vi "Remove Indentation.vi"(10 "levels to remove":i32, 11 "String in":string) -> (3 "String":string)   [LabVIEW 2013]
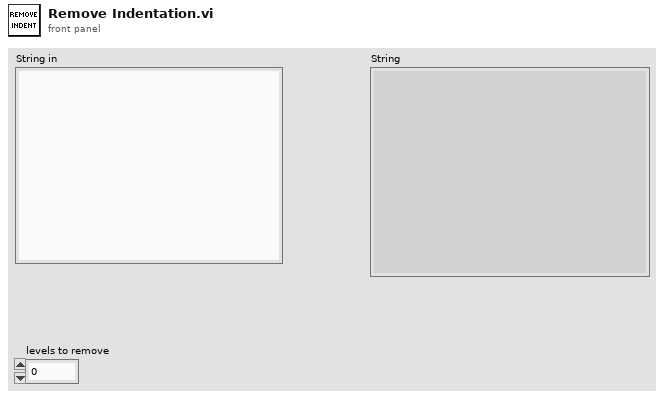
[diagram p1: front panel]
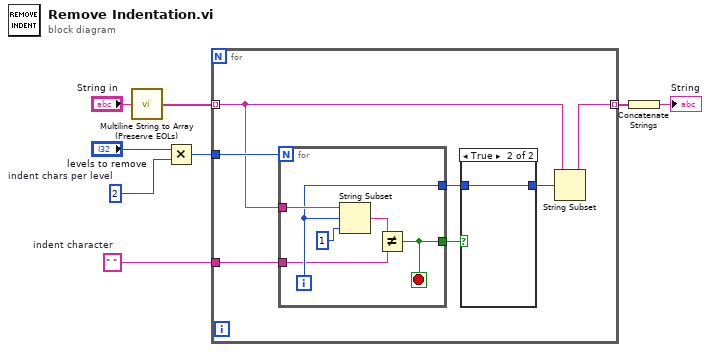
[diagram p0: block diagram]
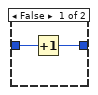
[diagram p2: hidden frame]
diagram:
  w1 = " "  # indent character
  w5 = 2  # indent chars per level
  n1 = call "Multiline String to Array (Preserve EOLs).vi"("Input String"="String in") -> ("Array"=w7:string[])
  n2 = Multiply(x="levels to remove", y=w5) -> (x*y=w4:i32)
  n3 = for {
    tunnel: w7 -> [w14] mode=indexing
    tunnel: w4 -> [w15]
    tunnel: [w13] -> w3 mode=indexing
    tunnel: w1 -> [w9]
    n4 = for {
      N: w15 -> [_]
      tunnel: w14 -> [w24]
      tunnel: [w21] -> w10
      tunnel: [w20] -> w12
      tunnel: w9 -> [w19]
      i -> [w21]
      stop <- w20 stop-if-true
      n5 = String Subset(string=w24, offset (0)=w21, length (rest)=1 ("length (rest)")) -> (substring=w22:string)
      n6 = Not Equal?(x=w22, y=w19) -> (x != y?=w20:bool)
    }
    n7 = case shown="True" w12 {
      tunnel: [w16 w18] -> w11
      tunnel: w10 -> [w17 w18]
      frame False {
        n8 = Increment(x=w17) -> (x+1=w16:i32)
      }
      frame True {
      }
    }
    n9 = String Subset(string=w14, offset (0)=w11) -> (substring=w13:string)  [unwired: 1 in]
  }
  n10 = Concatenate Strings(w3) -> (→"String":string)
